vi "Build SHDLCCommand.vi"(9 "Data":u8[](array[numeric]) format="%x", 10 "CommandID":u8 format="%x", 11 "SlaveAdress":u8 format="%x") -> (3 "ByteArrayToSend":u8[](array[numeric]) format="%x")   [LabVIEW 2019]
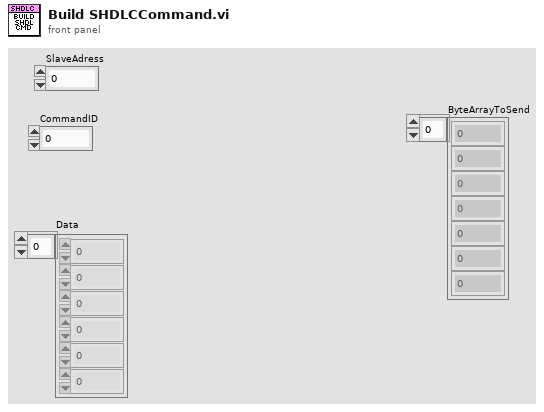
[diagram p1: front panel]
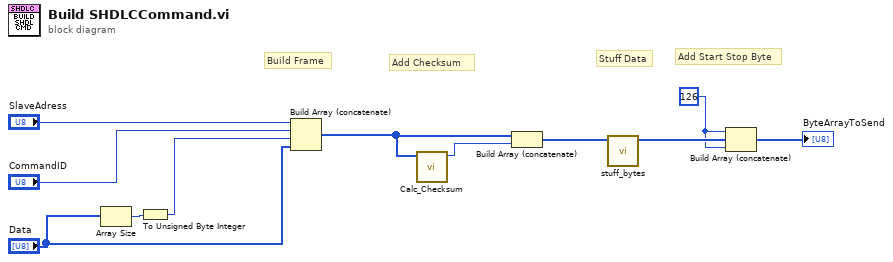
[diagram p0: block diagram]
diagram:
  w2 = u8 126 ("SlaveAdress")
  # "Add Start Stop Byte"
  # "Stuff Data"
  # "Add Checksum"
  # "Build Frame"
  n1 = Array Size(array="Data") -> (size(s)=w9:i32)
  n2 = To Unsigned Byte Integer(number=w9) -> (unsigned 8bit integer=w8:u8)
  n3 = Build Array (concatenate)("SlaveAdress", "CommandID", w8, "Data") -> (w6:u8[])
  n4 = call "Calc_Checksum.vi"("DataFrame"=w6) -> ("Checksum"=w5:u8)  [unwired: 10 in]
  n5 = Build Array (concatenate)(w6, w5) -> (w4:u8[])
  n6 = call "stuff_bytes.vi"("ByteArrayIn"=w4) -> ("StuffedDataOut"=w3:u8[])  [unwired: 10 in]
  n7 = Build Array (concatenate)(w2, w3, w2) -> (→"ByteArrayToSend":u8[])
